vi "DPO_7K_AskForATI.vi"(8 "Error In":errorcluster, 10 "Channel":u16(ring) items=["Channel 1", "Channel 2", "Channel 3", "Channel 4", "Math 1", "Math 2", "Math 3", "Math 4", "Reference 1", "Reference 2", "Reference 3", "Reference 4"], 11 "VISA resource name in":refnum<visa-resource-name>) -> (0 "Error Out":errorcluster, 2 "ATI?":bool, 3 "VISA resource name out":refnum<visa-resource-name>)   [LabVIEW 2020]
panel:
  out "concatenated string":string
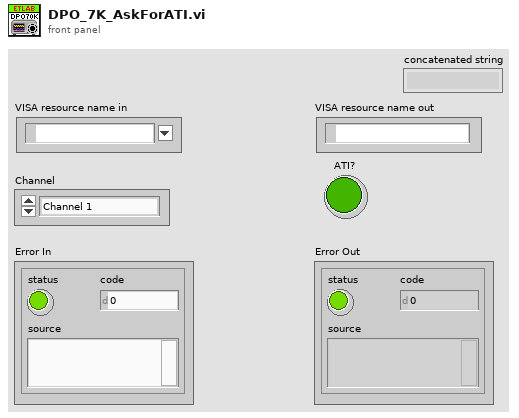
[diagram p1: front panel]
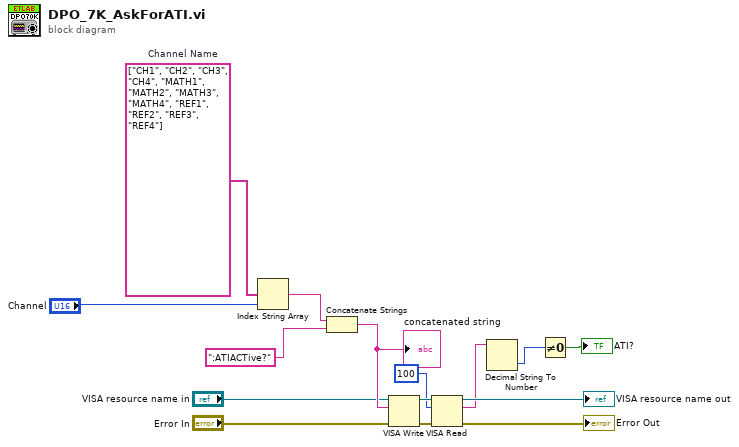
[diagram p0: block diagram]
diagram:
  w3 = string[] ["CH1", "CH2", "CH3", "CH4", "MATH1", "MATH2", "MATH3", "MATH4", "REF1", "REF2", "REF3", "REF4"]  # Channel Name
  n1 = Index String Array(1:"Channel", 2:w3) -> (0:w1:string)  [unwired: 1 in]
  n2 = Concatenate Strings(w1, ":ATIACTive?" ("write buffer")) -> (w14:string)
  "concatenated string" <- w14
  n3 = VISA Write(VISA resource name="VISA resource name in", write buffer=w14, error in (no error)="Error In") -> (VISA resource name out=w12:refnum<visa-resource-name>, error out=w13:errorcluster)  [unwired: 1 out]
  n4 = VISA Read(VISA resource name=w12, byte count=u32 100, error in (no error)=w13) -> (VISA resource name out=→"VISA resource name out":refnum<visa-resource-name>, read buffer=w5:string, error out=→"Error Out":errorcluster)  [unwired: 1 out]
  n5 = Decimal String To Number(string=w5) -> (number=w4:i32)  [unwired: 2 in, 1 out]
  n6 = Not Equal To 0?(x=w4) -> (x != 0?=→"ATI?":bool)
